vi "idle.vi"(7 "Def Set":dbl=50.0 caption="Default Setpoint (C)" format="%.2f") -> ()   [LabVIEW 2016]
doc: "This subvi sets up the global temperature controller subvis so that the temp controller will continue to keep the bug's temperature at a safe temperature for an indefinite time in between experiment executions.\n\nPaul K Dixon\nPhysics 350\nCSUSB Physics"
uses:
  temp control/globals/temp control global variables.vi
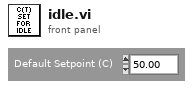
[diagram p1: front panel]
types:
  T1 = typedef "control parameters.ctl" = cluster{"Setpoint":dbl, "Control bandwidth":dbl, "Settle bandwidth":dbl, "Integral time":dbl, "Int\non":bool, "Derivative time":dbl, "Der\non":bool, "Settle time":dbl}
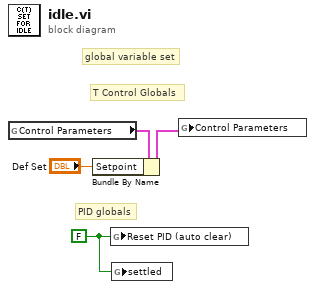
[diagram p0: block diagram]
diagram:
  w4 = FALSE ("Reset PID (auto clear)")
  # "PID globals"
  # "T Control Globals"
  # "global variable set"
  n1 = global read "temp control global variables.vi" "Control Parameters"() -> (w1:T1)
  n2 = Bundle By Name(cluster=w1, "Setpoint"="Def Set") -> (w2:T1)
  n3 = global write "temp control global variables.vi" "Reset PID (auto clear)"(w4) -> ()
  n4 = global write "temp control global variables.vi" "settled"(w4) -> ()
  n5 = global write "temp control global variables.vi" "Control Parameters"(w2) -> ()
